vi "Fdx Create Tx Queue.vi"(8 "error in (no error)":errorcluster, 10 "QueueSizeIn":u32, 11 "InstrumentHandle_port in":u32) -> (0 "error out":errorcluster, 2 "TxQueueInfo":cluster{"QueueBaseAddr":u32, "QueueSizeOut":u32}, 3 "InstrumentHandle_port out":u32)   [LabVIEW 2020, in "AIM664LV.lvlib"]
uses:
  AIM664LV.lvlib
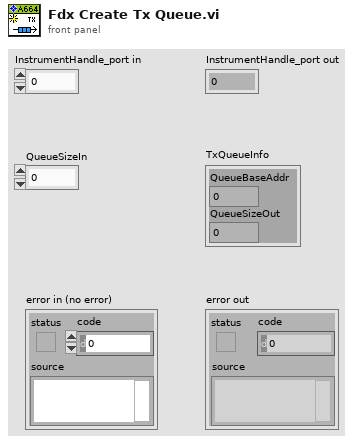
[diagram p1: front panel]
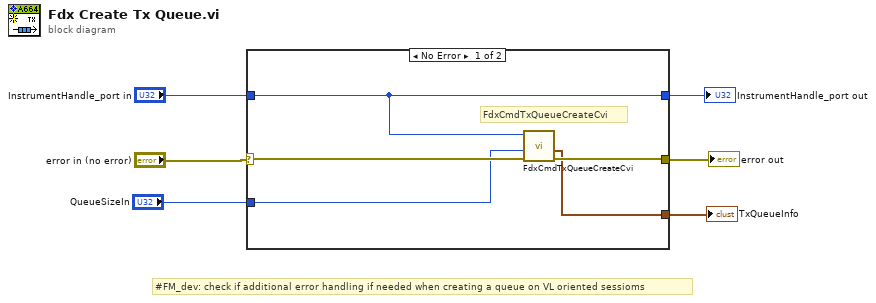
[diagram p0: block diagram]
diagram:
  # "#FM_dev: check if additional error handling if needed when creating a queue on VL oriented sessioms"
  n1 = case shown="No Error" "error in (no error)" {
    selector: "error in (no error)" -> [w11 w12]
    tunnel: "InstrumentHandle_port in" -> [w7 w13]
    tunnel: [w9 w12] -> w4
    tunnel: [w7 w13] -> w3
    tunnel: "QueueSizeIn" -> [w10 _]
    tunnel: [w8 _] -> w1
    frame No Error {
      # "FdxCmdTxQueueCreateCvi"
      n2 = call "FdxCmdTxQueueCreateCvi.vi"("error in"=w11, "QueueSizeIn"=w10, "InstrumentHandle_port"=w7) -> ("error out"=w9:errorcluster, "TxQueueInfo"=w8:cluster{"QueueBaseAddr":u32, "QueueSizeOut":u32})  [unwired: 6 in, 1 out]
    }
    frame Error {
    }
  }
  "error out" <- w4
  "InstrumentHandle_port out" <- w3
  "TxQueueInfo" <- w1
